vi "Tracepoint_CreateDataEvent.vi"(8 "error in (no error)":errorcluster, 9 "data event":T5, 10 "data":T1, 11 "Qbus":refnum<class "Qbus.lvclass">) -> (0 "error out":errorcluster)   [LabVIEW 2017, in "CmsDataEventCreator.lvlib"]
uses:
  <vilib>/addons/InsightCM/Devices/Shared/Cms/CmsDataEventCreator/CmsDataEventCreator.lvlib
  <vilib>/addons/Qbus/Qbus.lvclass
  <vilib>/addons/InsightCM/Devices/Shared/Cms/CmsDataEventCreator/controls/DataEventConfig.ctl
  <vilib>/addons/InsightCM/Devices/Shared/Cms/CmsDataEventCreator/controls/AcqParams.ctl
  <vilib>/addons/InsightCM/Devices/Shared/Common/DataAccumulator/controls/AccumulationSettings.ctl
  <vilib>/addons/InsightCM/Devices/Shared/Common/DataAccumulator/controls/accumulationType.ctl
  <vilib>/addons/InsightCM/Devices/Shared/Common/DVRBuffer/controls/BufferLocation.ctl
  <vilib>/addons/PointValueMap/controls/PointMap.ctl
  <vilib>/addons/InsightCM/Devices/Shared/Common/DataFlow/controls/Data.ctl
  <vilib>/addons/InsightCM/Utilities/DataAccessors/controls/wfmSGL_DVR.ctl
  <vilib>/addons/InsightCM/Devices/Shared/Common/DataFlow/controls/Type.ctl
  <vilib>/addons/TraceLogger/TraceLogger.lvlib
  <vilib>/addons/InsightCM/Devices/Shared/Common/DataAccumulator/DataAccumulator.lvlib
  <vilib>/addons/InsightCM/Devices/Shared/Common/DVRBuffer/DVRBuffer.lvlib
  <vilib>/addons/PointValueMap/PointValueMap.lvlib
  <vilib>/addons/InsightCM/Devices/Shared/Common/DataFlow/DataFlow.lvlib
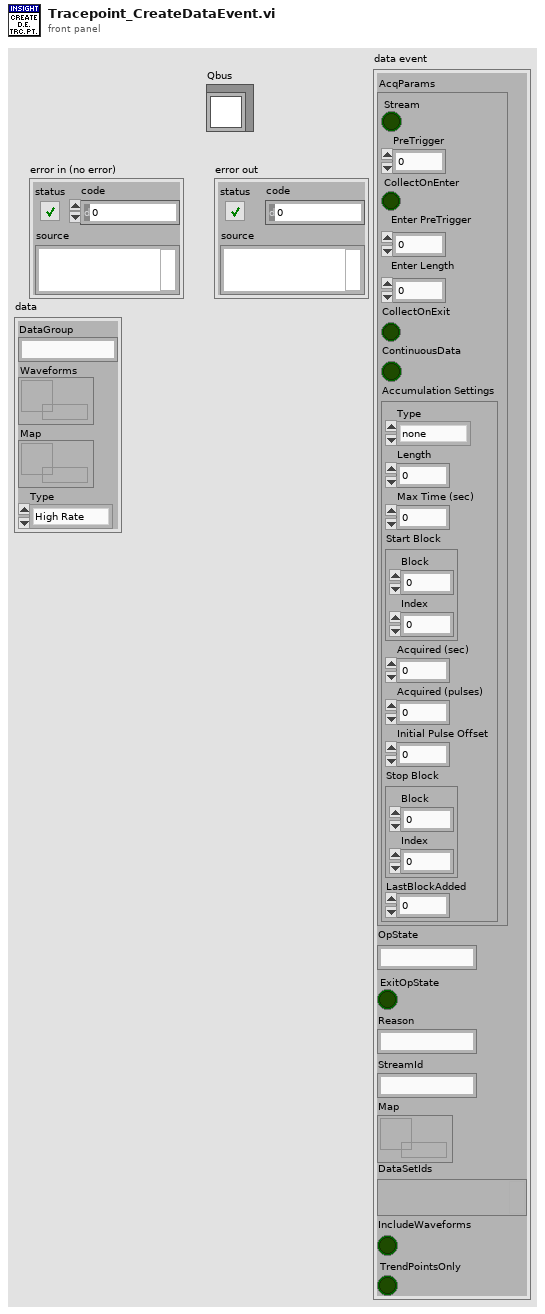
[diagram p1: front panel]
types:
  T1 = typedef "DataFlow.lvlib/Data.ctl" = cluster{"DataGroup":string, "Waveforms":T2, "Map":T3, "Type":T4}
  T2 = typedef "wfmSGL_DVR.ctl" = refnum<data-value>
  T3 = typedef "PointValueMap.lvlib/PointMap.ctl" = refnum<data-value>
  T4 = typedef "DataFlow.lvlib/Type.ctl" = enum16{"High Rate", "Low Rate", "Burst Mode"}
  T5 = typedef "CmsDataEventCreator.lvlib/DataEventConfig.ctl" = cluster{"AcqParams":T6, "OpState":string, "ExitOpState":bool, "Reason":string, "StreamId":string, "Map":T3, "DataSetIds":variant, "IncludeWaveforms":bool, "TrendPointsOnly":bool}
  T6 = typedef "CmsDataEventCreator.lvlib/AcqParams.ctl" = cluster{"Stream":bool, "PreTrigger":i32, "CollectOnEnter":bool, "Enter PreTrigger":i32, "Enter Length":dbl, "CollectOnExit":bool, "ContinuousData":bool, "Accumulation Settings":T7}
  T7 = typedef "DataAccumulator.lvlib/AccumulationSettings.ctl" = cluster{"Type":T8, "Length":dbl, "Max Time (sec)":dbl, "Start Block":T9, "Acquired (sec)":dbl, "Acquired (pulses)":i32, "Initial Pulse Offset":dbl, "Stop Block":T9, "LastBlockAdded":u32}
  T8 = typedef "DataAccumulator.lvlib/accumulationType.ctl" = enum16{"none", "seconds", "revolutions"}
  T9 = typedef "DVRBuffer.lvlib/BufferLocation.ctl" = cluster{"Block":u32, "Index":i32}
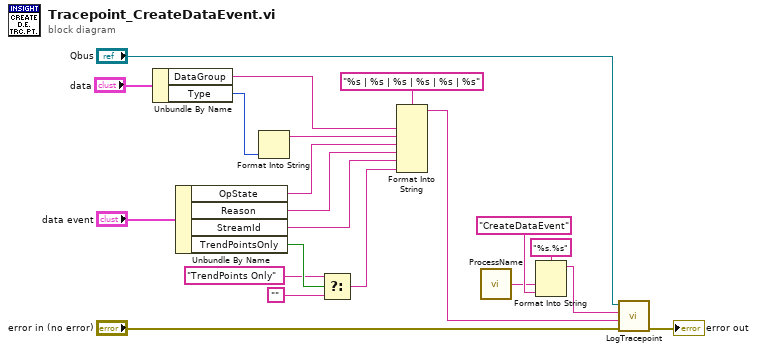
[diagram p0: block diagram]
diagram:
  n1 = Unbundle By Name("data") -> ("DataGroup"=w3:string, "Type"=w1:T4)
  n2 = Unbundle By Name("data event") -> ("OpState"=w5:string, "Reason"=w13:string, "StreamId"=w10:string, "TrendPointsOnly"=w9:bool)
  n3 = Format Into String(w1) -> (resulting string=w2:string)  [unwired: 3 in, 1 out]
  n4 = Select(t="TrendPoints Only" ("StreamId"), s=w9, f="") -> (s? t:f=w7:string)
  n5 = Format Into String(format string="%s | %s | %s | %s | %s | %s", w3, w2, w5, w13, w10, w7) -> (resulting string=w12:string)  [unwired: 2 in, 1 out]
  n6 = call <vilib>:"ProcessName.vi"() -> ("process name"=w15:string)  [unwired: 5 in]
  n7 = Format Into String(format string="%s.%s", w15, "CreateDataEvent" ("tracepoint")) -> (resulting string=w17:string)  [unwired: 2 in, 1 out]
  n8 = call <vilib>:"LogTracepoint.vi"("error in (no error)"="error in (no error)", "log string"=w12, "tracepoint"=w17, "qbus in"="Qbus") -> ("error out"=→"error out":errorcluster)  [unwired: 6 in, 1 out]
